vi "Create 4 In 4 Out Channel Resources.vi"(0 "common resources":T9={"sync pulse resources"={"sync pulse destination terminal"="", "sync100"="", "sync pulse source terminal"="", "imported sync pulse register"="", "generate sync pulse handshake"="", "enable sync pulse register"="", "sync pulse clock"=""}, "serial channel resources"={"sc 0"={"completed frames register"=""}, "sc 1"={"completed frames register"=""}, "sc 2"={"completed frames register"=""}, "sc 3"={"completed frames register"=""}, "sc 4"={"completed frames register"=""}, "sc 5"={"completed frames register"=""}, "sc 6"={"completed frames register"=""}, "sc 7"={"completed frames register"=""}}, "dram manager 0"={"DRAM class"=refnum, "process clock"="", "registers"={"configuration"={"write time slice"="", "request time slice"="", "DRAM arbiter config"="", "partition config"=""}, "reset"={"handshake"={"start.go"="", "start.go rcvd"="", "done.go"="", "done.go rcvd"=""}, "process"={"in"="", "out"=""}, "write"={"in"="", "out 0"="", "out 1"="", "out 2"="", "out 3"=""}, "read"={"in"="", "out 0"="", "out 1"="", "out 2"="", "out 3"=""}}, "status"={"partition full"=""}}, "FIFOs"={"write data"={"FIFO 0"="", "FIFO 1"="", "FIFO 2"="", "FIFO 3"=""}, "request metadata"={"FIFO"=""}, "read data VOQ"={"FIFO 0"="", "FIFO 1"="", "FIFO 2"="", "FIFO 3"=""}, "read data"={"FIFO 0"="", "FIFO 1"="", "FIFO 2"="", "FIFO 3"=""}}, "num active streams"=0.0, "max open read requests"=256}, "dram manager 1"={"DRAM class"=refnum, "process clock"="", "registers"={"configuration"={"write time slice"="", "request time slice"="", "DRAM arbiter config"="", "partition config"=""}, "reset"={"handshake"={"start.go"="", "start.go rcvd"="", "done.go"="", "done.go rcvd"=""}, "process"={"in"="", "out"=""}, "write"={"in"="", "out 0"="", "out 1"="", "out 2"="", "out 3"=""}, "read"={"in"="", "out 0"="", "out 1"="", "out 2"="", "out 3"=""}}, "status"={"partition full"=""}}, "FIFOs"={"write data"={"FIFO 0"="", "FIFO 1"="", "FIFO 2"="", "FIFO 3"=""}, "request metadata"={"FIFO"=""}, "read data VOQ"={"FIFO 0"="", "FIFO 1"="", "FIFO 2"="", "FIFO 3"=""}, "read data"={"FIFO 0"="", "FIFO 1"="", "FIFO 2"="", "FIFO 3"=""}}, "num active streams"=0.0, "max open read requests"=256}}) -> (4 "channel resources":T1)   [LabVIEW 2020, in "GettingStarted_Gen_148X_FPGA.lvlib"]
uses:
  GettingStarted_Gen_148X_FPGA.lvlib
  Common/Types/Common Resources.ctl
  <instrlib>/_niInstr/Memory/v1/FPGA/DRAM/niInstr Memory DRAM v1 FPGA.lvclass
  <instrlib>/FlexRIO/CSI-2/v2/FPGA/Types/Sync Pulse Resources.ctl
  Common/Types/Serial Channel Resources.ctl
  Common/Types/Single Serial Channel Resources.ctl
  <instrlib>/FlexRIO/CSI-2/v2/FPGA/DRAM Manager/Private/DRAM Manager.ctl
  <instrlib>/FlexRIO/CSI-2/v2/FPGA/DRAM Manager/Private/Common/DRAM Manager Registers.ctl
  <instrlib>/FlexRIO/CSI-2/v2/FPGA/DRAM Manager/Private/Common/Handshake Registers.ctl
  <instrlib>/FlexRIO/CSI-2/v2/FPGA/DRAM Manager/Private/Common/DRAM Manager FIFOs.ctl
  <instrlib>/FlexRIO/CSI-2/v2/FPGA/DRAM Manager/Private/Common/Write Data FIFO Ref.ctl
  <instrlib>/FlexRIO/CSI-2/v2/FPGA/DRAM Manager/Private/Common/Read Request Metadata FIFO Ref.ctl
  <instrlib>/FlexRIO/CSI-2/v2/FPGA/DRAM Manager/Private/Common/Read Data FIFO Ref.ctl
  Types/4 In 4 Out Channel Resources.ctl
  Types/Serial Output Channel Resources.ctl
  Common/Types/Serial Output Channel IO.ctl
  Common/Types/Serial Output Channel IO 32b.ctl
  Common/Types/Serial Output Channel IO 64b.ctl
  Common/Types/I2C IO.ctl
  Types/Serial Input Channel Resources.ctl
  Common/GettingStarted_Common_148X_FPGA.lvlib
  <instrlib>/FlexRIO/CSI-2/v2/FPGA/DRAM Manager/DRAM Manager v2.lvlib
  <instrlib>/FlexRIO/CSI-2/v2/FPGA/NI CSI-2 API FPGA v2.lvlib
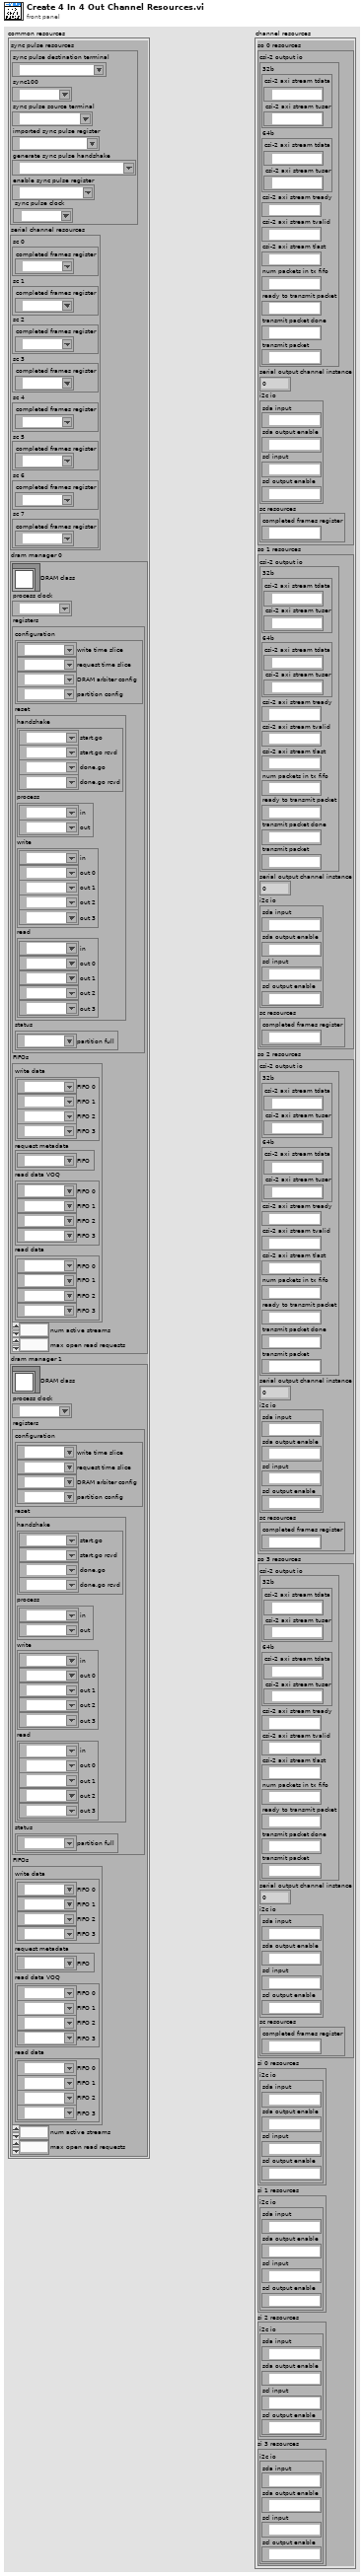
[diagram p1: front panel]
types:
  T1 = typedef "GettingStarted_Gen_148X_FPGA.lvlib/4 In 4 Out Channel Resources.ctl" = cluster{"so 0 resources":T2, "so 1 resources":T2, "so 2 resources":T2, "so 3 resources":T2, "si 0 resources":T8, "si 1 resources":T8, "si 2 resources":T8, "si 3 resources":T8}
  T2 = typedef "GettingStarted_Gen_148X_FPGA.lvlib/Serial Output Channel Resources.ctl" = cluster{"csi-2 output io":T3, "serial output channel instance":u8, "i2c io":T6, "sc resources":T7}
  T3 = typedef "GettingStarted_Common_148X_FPGA.lvlib/Serial Output Channel IO.ctl" = cluster{"32b":T4, "64b":T5, "csi-2 axi stream tready":refnum<k21>, "csi-2 axi stream tvalid":refnum<k21>, "csi-2 axi stream tlast":refnum<k21>, "num packets in tx fifo":refnum<k21>, "ready to transmit packet":refnum<k21>, "transmit packet done":refnum<k21>, "transmit packet":refnum<k21>}
  T4 = typedef "GettingStarted_Common_148X_FPGA.lvlib/Serial Output Channel IO 32b.ctl" = cluster{"csi-2 axi stream tdata":refnum<k21>, "csi-2 axi stream tuser":refnum<k21>}
  T5 = typedef "GettingStarted_Common_148X_FPGA.lvlib/Serial Output Channel IO 64b.ctl" = cluster{"csi-2 axi stream tdata":refnum<k21>, "csi-2 axi stream tuser":refnum<k21>}
  T6 = typedef "GettingStarted_Common_148X_FPGA.lvlib/I2C IO.ctl" = cluster{"sda input":refnum<k21>, "sda output enable":refnum<k21>, "scl input":refnum<k21>, "scl output enable":refnum<k21>}
  T7 = typedef "GettingStarted_Common_148X_FPGA.lvlib/Single Serial Channel Resources.ctl" = cluster{"completed frames register":refnum<k21>}
  T8 = typedef "GettingStarted_Gen_148X_FPGA.lvlib/Serial Input Channel Resources.ctl" = cluster{"i2c io":T6}
  T9 = typedef "GettingStarted_Common_148X_FPGA.lvlib/Common Resources.ctl" = cluster{"sync pulse resources":T10, "serial channel resources":T11, "dram manager 0":T12, "dram manager 1":T12}
  T10 = typedef "NI CSI-2 API FPGA v2.lvlib/Sync Pulse Resources.ctl" = cluster{"sync pulse destination terminal":refnum<k21>, "sync100":refnum<k21>, "sync pulse source terminal":refnum<k21>, "imported sync pulse register":refnum<k21>, "generate sync pulse handshake":refnum<k21>, "enable sync pulse register":refnum<k21>, "sync pulse clock":refnum<k21>}
  T11 = typedef "GettingStarted_Common_148X_FPGA.lvlib/Serial Channel Resources.ctl" = cluster{"sc 0":T7, "sc 1":T7, "sc 2":T7, "sc 3":T7, "sc 4":T7, "sc 5":T7, "sc 6":T7, "sc 7":T7}
  T12 = typedef "DRAM Manager v2.lvlib/DRAM Manager.ctl" = cluster{"DRAM class":refnum<class "niInstr Memory DRAM v1 FPGA.lvclass">, "process clock":refnum<k21>, "registers":T13, "FIFOs":T15, "num active streams":fxp<+,3,3>, "max open read requests":u16}
  T13 = typedef "DRAM Manager v2.lvlib/DRAM Manager Registers.ctl" = cluster{"configuration":cluster{"write time slice":refnum<k21>, "request time slice":refnum<k21>, "DRAM arbiter config":refnum<k21>, "partition config":refnum<k21>}, "reset":cluster{"handshake":T14, "process":cluster{"in":refnum<k21>, "out":refnum<k21>}, "write":cluster{"in":refnum<k21>, "out 0":refnum<k21>, "out 1":refnum<k21>, "out 2":refnum<k21>, "out 3":refnum<k21>}, "read":cluster{"in":refnum<k21>, "out 0":refnum<k21>, "out 1":refnum<k21>, "out 2":refnum<k21>, "out 3":refnum<k21>}}, "status":cluster{"partition full":refnum<k21>}}
  T14 = typedef "DRAM Manager v2.lvlib/Handshake Registers.ctl" = cluster{"start.go":refnum<k21>, "start.go rcvd":refnum<k21>, "done.go":refnum<k21>, "done.go rcvd":refnum<k21>}
  T15 = typedef "DRAM Manager v2.lvlib/DRAM Manager FIFOs.ctl" = cluster{"write data":cluster{"FIFO 0":T16, "FIFO 1":T16, "FIFO 2":T16, "FIFO 3":T16}, "request metadata":cluster{"FIFO":T17}, "read data VOQ":cluster{"FIFO 0":T18, "FIFO 1":T18, "FIFO 2":T18, "FIFO 3":T18}, "read data":cluster{"FIFO 0":T18, "FIFO 1":T18, "FIFO 2":T18, "FIFO 3":T18}}
  T16 = typedef "DRAM Manager v2.lvlib/Write Data FIFO Ref.ctl" = refnum<k21>
  T17 = typedef "DRAM Manager v2.lvlib/Read Request Metadata FIFO Ref.ctl" = refnum<k21>
  T18 = typedef "DRAM Manager v2.lvlib/Read Data FIFO Ref.ctl" = refnum<k21>
  T19 = cluster{"serial output 0 io":T3, "serial output 1 io":T3, "serial output 2 io":T3, "serial output 3 io":T3}
  T20 = cluster{"serial output 2 i2c io":T6, "serial output 1 i2c io":T6, "serial output 0 i2c io":T6, "serial output 3 i2c io":T6}
  T21 = cluster{"serial input 0 i2c io":T6, "serial input 1 i2c io":T6, "serial input 2 i2c io":T6, "serial input 3 i2c io":T6}
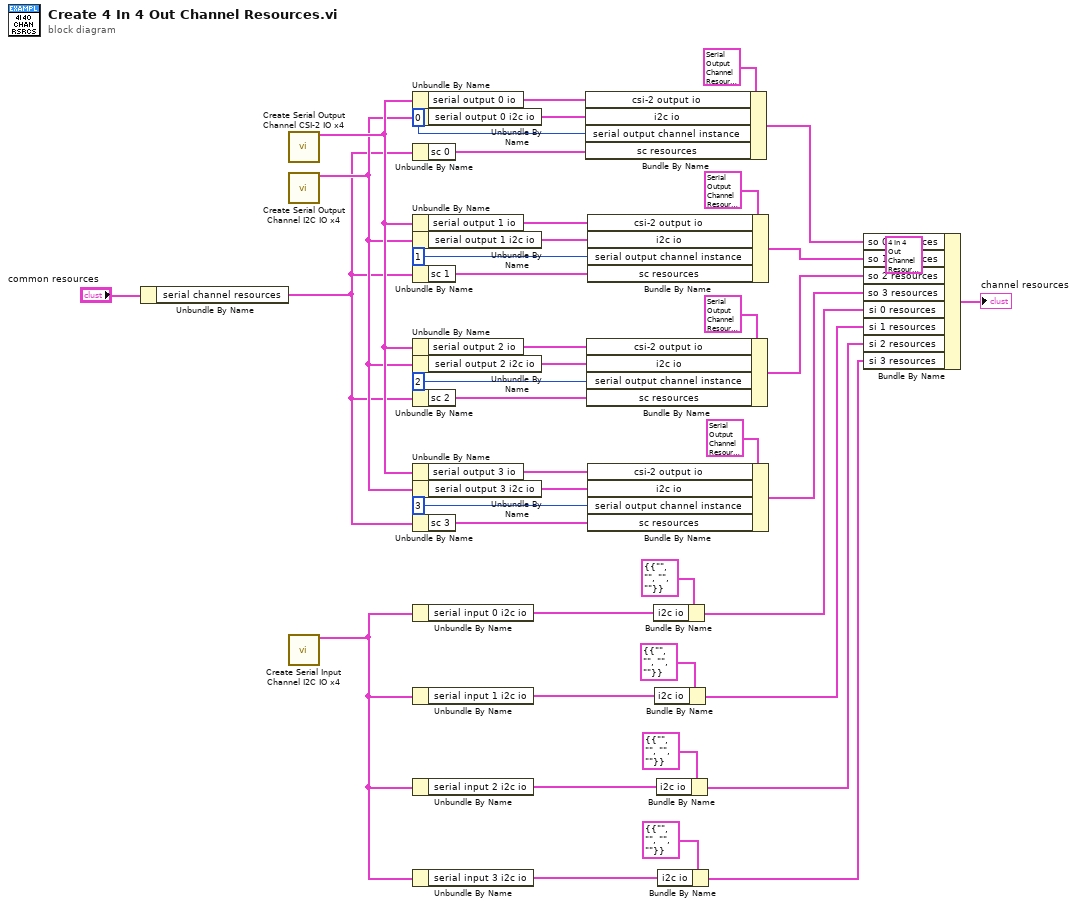
[diagram p0: block diagram]
diagram:
  n1 = Unbundle By Name("common resources") -> ("serial channel resources"=w12:T11)
  n2 = call "Create Serial Output Channel CSI-2 IO x4.vi"() -> ("serial output channel csi-2 io x4 2"=w22:T19)  [unwired: 15 in]
  n3 = call "Create Serial Output Channel I2C IO x4.vi"() -> ("serial output channel i2c io x4"=w21:T20)  [unwired: 15 in]
  n4 = call "Create Serial Input Channel I2C IO x4.vi"() -> ("serial input channel i2c io x4"=w11:T21)  [unwired: 15 in]
  n5 = Unbundle By Name(w22) -> ("serial output 0 io"=w23:T3)
  n6 = Unbundle By Name(w21) -> ("serial output 0 i2c io"=w34:T6)
  n7 = Unbundle By Name(w12) -> ("sc 0"=w16:T7)
  n8 = Unbundle By Name(w22) -> ("serial output 1 io"=w33:T3)
  n9 = Unbundle By Name(w21) -> ("serial output 1 i2c io"=w32:T6)
  n10 = Unbundle By Name(w12) -> ("sc 1"=w15:T7)
  n11 = Unbundle By Name(w22) -> ("serial output 2 io"=w31:T3)
  n12 = Unbundle By Name(w21) -> ("serial output 2 i2c io"=w30:T6)
  n13 = Unbundle By Name(w12) -> ("sc 2"=w14:T7)
  n14 = Unbundle By Name(w22) -> ("serial output 3 io"=w29:T3)
  n15 = Unbundle By Name(w21) -> ("serial output 3 i2c io"=w28:T6)
  n16 = Unbundle By Name(w12) -> ("sc 3"=w13:T7)
  n17 = Unbundle By Name(w11) -> ("serial input 0 i2c io"=w27:T6)
  n18 = Unbundle By Name(w11) -> ("serial input 1 i2c io"=w26:T6)
  n19 = Unbundle By Name(w11) -> ("serial input 2 i2c io"=w25:T6)
  n20 = Unbundle By Name(w11) -> ("serial input 3 i2c io"=w24:T6)
  n21 = Bundle By Name(cluster=T2 {"csi-2 output io"={"32b"={"csi-2 axi stream tdata"="", "csi-2 axi stream tuser"=""}, "64b"={"csi-2 axi stream tdata"="", "csi-2 axi stream tuser"=""}, "csi-2 axi stream tready"="", "csi-2 axi stream tvalid"="", "csi-2 axi stream tlast"="", "num packets in tx fifo"="", "ready to transmit packet"="", "transmit packet done"="", "transmit packet"=""}, "serial output channel instance"=0, "i2c io"={"sda input"="", "sda output enable"="", "scl input"="", "scl output enable"=""}, "sc resources"={"completed frames register"=""}} ("si 0 resources"), "csi-2 output io"=w23, "i2c io"=w34, "serial output channel instance"=u8 0 ("serial input channel instance"), "sc resources"=w16) -> (w41:T2)
  n22 = Bundle By Name(cluster=T2 {"csi-2 output io"={"32b"={"csi-2 axi stream tdata"="", "csi-2 axi stream tuser"=""}, "64b"={"csi-2 axi stream tdata"="", "csi-2 axi stream tuser"=""}, "csi-2 axi stream tready"="", "csi-2 axi stream tvalid"="", "csi-2 axi stream tlast"="", "num packets in tx fifo"="", "ready to transmit packet"="", "transmit packet done"="", "transmit packet"=""}, "serial output channel instance"=0, "i2c io"={"sda input"="", "sda output enable"="", "scl input"="", "scl output enable"=""}, "sc resources"={"completed frames register"=""}} ("si 0 resources"), "csi-2 output io"=w31, "i2c io"=w30, "serial output channel instance"=u8 2 ("serial input channel instance"), "sc resources"=w14) -> (w37:T2)
  n23 = Bundle By Name(cluster=T2 {"csi-2 output io"={"32b"={"csi-2 axi stream tdata"="", "csi-2 axi stream tuser"=""}, "64b"={"csi-2 axi stream tdata"="", "csi-2 axi stream tuser"=""}, "csi-2 axi stream tready"="", "csi-2 axi stream tvalid"="", "csi-2 axi stream tlast"="", "num packets in tx fifo"="", "ready to transmit packet"="", "transmit packet done"="", "transmit packet"=""}, "serial output channel instance"=0, "i2c io"={"sda input"="", "sda output enable"="", "scl input"="", "scl output enable"=""}, "sc resources"={"completed frames register"=""}} ("si 0 resources"), "csi-2 output io"=w33, "i2c io"=w32, "serial output channel instance"=u8 1 ("serial input channel instance"), "sc resources"=w15) -> (w39:T2)
  n24 = Bundle By Name(cluster=T2 {"csi-2 output io"={"32b"={"csi-2 axi stream tdata"="", "csi-2 axi stream tuser"=""}, "64b"={"csi-2 axi stream tdata"="", "csi-2 axi stream tuser"=""}, "csi-2 axi stream tready"="", "csi-2 axi stream tvalid"="", "csi-2 axi stream tlast"="", "num packets in tx fifo"="", "ready to transmit packet"="", "transmit packet done"="", "transmit packet"=""}, "serial output channel instance"=0, "i2c io"={"sda input"="", "sda output enable"="", "scl input"="", "scl output enable"=""}, "sc resources"={"completed frames register"=""}} ("si 0 resources"), "csi-2 output io"=w29, "i2c io"=w28, "serial output channel instance"=u8 3 ("serial input channel instance"), "sc resources"=w13) -> (w35:T2)
  n25 = Bundle By Name(cluster=T8 {"i2c io"={"sda input"="", "sda output enable"="", "scl input"="", "scl output enable"=""}} ("si 0 resources"), "i2c io"=w27) -> (w5:T8)
  n26 = Bundle By Name(cluster=T8 {"i2c io"={"sda input"="", "sda output enable"="", "scl input"="", "scl output enable"=""}} ("si 0 resources"), "i2c io"=w26) -> (w4:T8)
  n27 = Bundle By Name(cluster=T8 {"i2c io"={"sda input"="", "sda output enable"="", "scl input"="", "scl output enable"=""}} ("si 0 resources"), "i2c io"=w25) -> (w3:T8)
  n28 = Bundle By Name(cluster=T8 {"i2c io"={"sda input"="", "sda output enable"="", "scl input"="", "scl output enable"=""}} ("si 0 resources"), "i2c io"=w24) -> (w2:T8)
  n29 = Bundle By Name(cluster=T1 {"so 0 resources"={"csi-2 output io"={"32b"={"csi-2 axi stream tdata"="", "csi-2 axi stream tuser"=""}, "64b"={"csi-2 axi stream tdata"="", "csi-2 axi stream tuser"=""}, "csi-2 axi stream tready"="", "csi-2 axi stream tvalid"="", "csi-2 axi stream tlast"="", "num packets in tx fifo"="", "ready to transmit packet"="", "transmit packet done"="", "transmit packet"=""}, "serial output channel instance"=0, "i2c io"={"sda input"="", "sda output enable"="", "scl input"="", "scl output enable"=""}, "sc resources"={"completed frames register"=""}}, "so 1 resources"={"csi-2 output io"={"32b"={"csi-2 axi stream tdata"="", "csi-2 axi stream tuser"=""}, "64b"={"csi-2 axi stream tdata"="", "csi-2 axi stream tuser"=""}, "csi-2 axi stream tready"="", "csi-2 axi stream tvalid"="", "csi-2 axi stream tlast"="", "num packets in tx fifo"="", "ready to transmit packet"="", "transmit packet done"="", "transmit packet"=""}, "serial output channel instance"=0, "i2c io"={"sda input"="", "sda output enable"="", "scl input"="", "scl output enable"=""}, "sc resources"={"completed frames register"=""}}, "so 2 resources"={"csi-2 output io"={"32b"={"csi-2 axi stream tdata"="", "csi-2 axi stream tuser"=""}, "64b"={"csi-2 axi stream tdata"="", "csi-2 axi stream tuser"=""}, "csi-2 axi stream tready"="", "csi-2 axi stream tvalid"="", "csi-2 axi stream tlast"="", "num packets in tx fifo"="", "ready to transmit packet"="", "transmit packet done"="", "transmit packet"=""}, "serial output channel instance"=0, "i2c io"={"sda input"="", "sda output enable"="", "scl input"="", "scl output enable"=""}, "sc resources"={"completed frames register"=""}}, "so 3 resources"={"csi-2 output io"={"32b"={"csi-2 axi stream tdata"="", "csi-2 axi stream tuser"=""}, "64b"={"csi-2 axi stream tdata"="", "csi-2 axi stream tuser"=""}, "csi-2 axi stream tready"="", "csi-2 axi stream tvalid"="", "csi-2 axi stream tlast"="", "num packets in tx fifo"="", "ready to transmit packet"="", "transmit packet done"="", "transmit packet"=""}, "serial output channel instance"=0, "i2c io"={"sda input"="", "sda output enable"="", "scl input"="", "scl output enable"=""}, "sc resources"={"completed frames register"=""}}, "si 0 resources"={"i2c io"={"sda input"="", "sda output enable"="", "scl input"="", "scl output enable"=""}}, "si 1 resources"={"i2c io"={"sda input"="", "sda output enable"="", "scl input"="", "scl output enable"=""}}, "si 2 resources"={"i2c io"={"sda input"="", "sda output enable"="", "scl input"="", "scl output enable"=""}}, "si 3 resources"={"i2c io"={"sda input"="", "sda output enable"="", "scl input"="", "scl output enable"=""}}} ("so channel resources 2"), "so 0 resources"=w41, "so 1 resources"=w39, "so 2 resources"=w37, "so 3 resources"=w35, "si 0 resources"=w5, "si 1 resources"=w4, "si 2 resources"=w3, "si 3 resources"=w2) -> (→"channel resources":T1)
